vi "Image_Handler.vi"(0 "Camera":T5, 5 "Data":T2={"L16 Linear Actuator"="", "XE 1000 Pump"="", "Camera1"="", "Camera2"="", "Camera1_IMG"=refnum, "Camera2_IMG"=refnum, "Img_Capt"=FALSE, "Actuator"=FALSE, "Pump"=FALSE, "Cam 1"=FALSE, "Cam 2"=FALSE, "Empty_Refill"=FALSE, "Crop"=FALSE, "Light intensity"=100, "Exposure Time"=1000.0, "Sample Name"="Test Sample", "Operator"="MRJ", "Calibration 1"=path "C:/Users/au540322/Desktop/IHS_Project/images/Debris/Debris_0/Debris_0_2019_06_01-23-32-49-686.PNG", "Calibration 2"=path "C:/Users/au540322/Desktop/IHS_Project/images/Debris/Debris_0/Debris_0_2019_06_01-23-32-49-686.PNG", "Framerate"=1, "Timeout Sample"=0, "Collection date"="MRJ", "Sample size threshold"=1, "Empty start"=1, "Command"="MRJ", "Calibration Image 1"=refnum, "Calibration Image 2"=refnum, "Original Image 1"=refnum, "Original Image 2"=refnum, "Processing Image 1"=refnum, "Processing Image 2"=refnum, "Object Image 1"=refnum, "Object Image 2"=refnum, "Cam 1 - save queue"=refnum, "Cam 2 - save queue"=refnum, "Station"="", "Species Name"="", "Other Notes"="", "Aperture"=enum."Item 0", "Image Process Queue Size"=500, "Image Save Queue Size"=500, "Overload threshold"=500, "Max Framerate"=100, "Blue Plane Image"=refnum, "Subtract Image"=refnum, "Binary Image 1"=refnum, "ROI mask allocation"=refnum, "Rectangle 1"={"Left"=0, "Top"=0, "Right"=0, "Bottom"=0, "Rotation"=0.0}, "Rectangle 2"={"Left"=0, "Top"=0, "Right"=0, "Bottom"=0, "Rotation"=0.0}, "Binary Image 2"=refnum, "Detection Region %"=0.0, "Cam 1 queue"=refnum, "Cam 2 queue"=refnum, "Detect image 1"=refnum, "Detect image 2"=refnum, "Detect 1"=path "C:/Users/au540322/Desktop/IHS_Project/images/Debris/Debris_0/Debris_0_2019_06_01-23-32-49-686.PNG", "Detect 2"=path "C:/Users/au540322/Desktop/IHS_Project/images/Debris/Debris_0/Debris_0_2019_06_01-23-32-49-686.PNG", "Max large object threshold"=0, "Open(T)/Close(F)"=FALSE} {"Rectangle 2"."Rotation" format="%.2f"; "Rectangle 2"."Left" scale=0.0..1024.0; "Rectangle 2"."Right" scale=0.0..1024.0; "Rectangle 1"."Rotation" format="%.2f"; "Rectangle 1"."Left" scale=0.0..1024.0; "Rectangle 1"."Right" scale=0.0..1024.0; "Max Framerate" min=1; "Overload threshold" min=1; "Image Save Queue Size" min=1; "Image Process Queue Size" min=1; "Empty start" min=1; "Sample size threshold" min=1; "Framerate" min=1; "Light intensity" scale=0.0..100.0}, 9 "Prev. sample":dbl, 11 "Timeout in":i32) -> (3 "Object":bool, 4 "Detected object":T1, 6 "Image Out":T1, 8 "Binary":T1, 10 "Sample nr":dbl, 15 "Timeout out":i32)   [LabVIEW 2019]
uses:
  Camera_ID.ctl
  controls/Data.ctl
  <vilib>/userdefined/High Color/IMAQdx.ctl
  <vilib>/vision/Image Controls.llb/IMAQ Image.ctl
panel:
  out "error out 1":errorcluster
  out "error out 2":errorcluster
  in  "error in":errorcluster
  out "error out":errorcluster
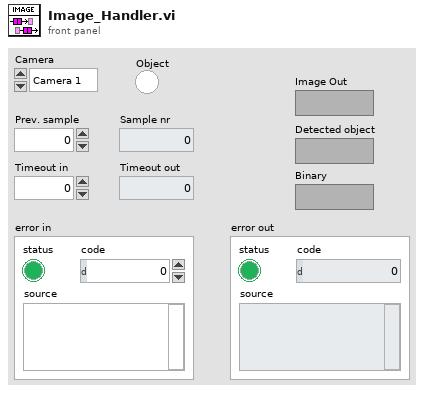
[diagram p1: front panel]
types:
  T1 = typedef "IMAQ Image.ctl" = refnum<image>
  T2 = typedef "Data.ctl" = cluster{"L16 Linear Actuator":refnum<visa-resource-name>, "XE 1000 Pump":refnum<visa-resource-name>, "Camera1":T3, "Camera2":T3, "Camera1_IMG":T1, "Camera2_IMG":T1, "Img_Capt":bool, "Actuator":bool, "Pump":bool, "Cam 1":bool, "Cam 2":bool, "Empty_Refill":bool, "Crop":bool, "Light intensity":i32, "Exposure Time":dbl, "Sample Name":string, "Operator":string, "Calibration 1":path, "Calibration 2":path, "Framerate":i32, "Timeout Sample":i32, "Collection date":string, "Sample size threshold":i32, "Empty start":u32, "Command":string, "Calibration Image 1":T1, "Calibration Image 2":T1, "Original Image 1":T1, "Original Image 2":T1, "Processing Image 1":T1, "Processing Image 2":T1, "Object Image 1":T1, "Object Image 2":T1, "Cam 1 - save queue":refnum<queue>, "Cam 2 - save queue":refnum<queue>, "Station":string, "Species Name":string, "Other Notes":string, "Aperture":enum32{"Item 0", "Item 1", "Item 2", "Item 3"}, "Image Process Queue Size":i32, "Image Save Queue Size":i32, "Overload threshold":i32, "Max Framerate":i32, "Blue Plane Image":T1, "Subtract Image":T1, "Binary Image 1":T1, "ROI mask allocation":T1, "Rectangle 1":T4, "Rectangle 2":T4, "Binary Image 2":T1, "Detection Region %":dbl, "Cam 1 queue":refnum<queue>, "Cam 2 queue":refnum<queue>, "Detect image 1":T1, "Detect image 2":T1, "Detect 1":path, "Detect 2":path, "Max large object threshold":i32, "Open(T)/Close(F)":bool}
  T3 = typedef "IMAQdx.ctl" = refnum<k21>
  T4 = typedef "IMAQ Rectangle" = cluster{"Left":i32, "Top":i32, "Right":i32, "Bottom":i32, "Rotation":dbl}
  T5 = typedef "Camera_ID.ctl" = enum16{"Camera 1", "Camera 2"}
  T6 = cluster{"Image Pixels (U32)":u32[][], "Checkbox":bool}
  T7 = cluster{"Timestamp":string, "Image Pixels (U32)":u32[][], "Prev. sample":dbl}
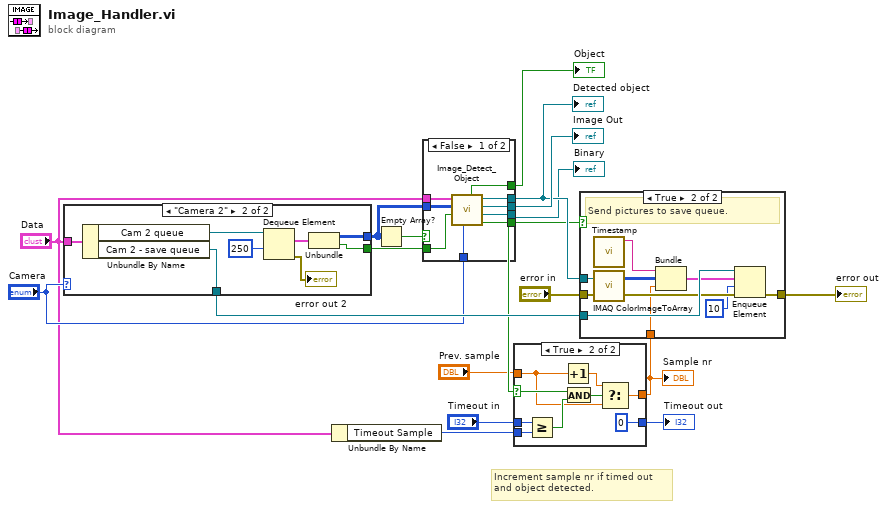
[diagram p0: block diagram]
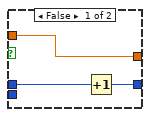
[diagram p2: hidden frame]
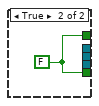
[diagram p4: hidden frame]
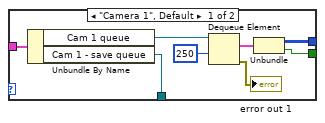
[diagram p5: hidden frame]
diagram:
  # "Increment sample nr if timed out \nand object detected."
  n1 = case shown="\"Camera 2\"" "Camera" {
    tunnel: "Data" -> [w26 w34]
    tunnel: [w21 w29] -> w15
    tunnel: [w20 w28] -> w6
    tunnel: [w19 w27] -> w1
    frame "Camera 1", Default {
      n2 = Unbundle By Name(w26) -> ("Cam 1 queue"=w24:refnum<queue>, "Cam 1 - save queue"=w21:refnum<queue>)
      n3 = Dequeue Element(queue=w24, timeout in ms (-1)=250) -> (element=w23:T6, error out=→"error out 1":errorcluster)  [unwired: 1 in, 2 out]
      n4 = Unbundle(w23) -> ("Image Pixels (U32)"=w20:u32[][], "Checkbox"=w19:bool)
    }
    frame "Camera 2" {
      n5 = Unbundle By Name(w34) -> ("Cam 2 queue"=w32:refnum<queue>, "Cam 2 - save queue"=w29:refnum<queue>)
      n6 = Dequeue Element(queue=w32, timeout in ms (-1)=250) -> (element=w31:T6, error out=→"error out 2":errorcluster)  [unwired: 1 in, 2 out]
      n7 = Unbundle(w31) -> ("Image Pixels (U32)"=w28:u32[][], "Checkbox"=w27:bool)
    }
  }
  n8 = Unbundle By Name("Data") -> ("Timeout Sample"=w8:i32)
  n9 = Empty Array?(array=w6) -> (empty?=w18:bool)
  n10 = case shown="False" w18 {
    tunnel: [w43 _] -> w16
    tunnel: [w42 w44] -> w11
    tunnel: "Data" -> [w41 _]
    tunnel: "Camera" -> [w40 _]
    tunnel: [w39 _] -> w17
    tunnel: w6 -> [w38 _]
    tunnel: [w37 _] -> w5
    tunnel: [w36 w44] -> w2
    tunnel: w1 -> [w35 _]
    frame False {
      n11 = call "Image_Detect_Object.vi"("Camera"=w40, "Detect Crop"=w35, "Image Pixels (U32)"=w38, "Data"=w41) -> ("Object accepted"=w42:bool, "Image Binary"=w37:T1, "New image"=w39:T1, "Crop Image Out"=w43:T1, "Object"=w36:bool)  [unwired: 3 in]
    }
    frame True {
      w44 = FALSE ("Object detected")
    }
  }
  "Detected object" <- w16
  "Image Out" <- w17
  "Binary" <- w5
  "Object" <- w2
  n12 = case shown="True" w11 {
    selector: w11 -> [_ w56]
    tunnel: w8 -> [_ w55]
    tunnel: [w47 0] -> w9
    tunnel: [w46 w50] -> w7
    tunnel: "Prev. sample" -> [w46 w49]
    tunnel: "Timeout in" -> [w45 w48]
    frame False {
      n13 = Increment(x=w45) -> (x+1=w47:i32)
    }
    frame True {
      n14 = Greater Or Equal?(x=w48, y=w55) -> (x >= y?=w54:bool)
      n15 = Increment(x=w49) -> (x+1=w51:dbl)
      n16 = And(x=w56, y=w54) -> (x .and. y?=w52:bool)
      n17 = Select(t=w51, s=w52, f=w49) -> (s? t:f=w50:dbl)
    }
  }
  "Sample nr" <- w7
  "Timeout out" <- w9
  n18 = case shown="True" w11 {
    tunnel: w16 -> [_ w67]
    tunnel: w15 -> [_ w66]
    tunnel: "error in" -> [w57 w65]
    tunnel: [w57 w63] -> w12
    tunnel: w7 -> [_ w59]
    frame False {
      # "No object within criteria."
    }
    frame True {
      # "Send pictures to save queue."
      n19 = call "Timestamp.vi"() -> ("Timestamp"=w60:string)  [unwired: 11 in]
      n20 = call "IMAQ ColorImageToArray"("Image"=w67, "error in (no error)"=w65) -> ("Image Pixels (U32)"=w61:u32[][], "error out"=w64:errorcluster)  [unwired: 2 in, 1 out]
      n21 = Bundle("Timestamp"=w60, "Image Pixels (U32)"=w61, "Prev. sample"=w59) -> (w62:T7)  [unwired: 1 in]
      n22 = Enqueue Element(queue=w66, element=w62, timeout in ms (-1)=10, error in (no error)=w64) -> (error out=w63:errorcluster)  [unwired: 2 out]
    }
  }
  "error out" <- w12
